vi "ChangePassword-Window.vi"(8 "error in (no error)":errorcluster, 11 "User Info":T1={"UserName"="", "Password"="", "Role"=enum."Admin"}) -> (0 "error out":errorcluster)   [LabVIEW 2017, in "Login-UI.lvlib"]
uses:
  Login-UI.lvlib
  User-Info.ctl
  User-Role.ctl
panel:
  in  "Cancel":bool
  in  "OK":bool
  in  "Password":string="admin" caption="密 码"
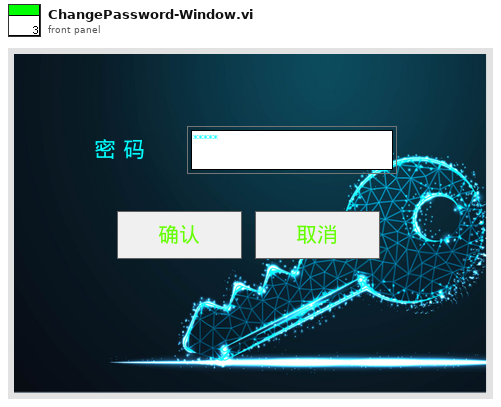
[diagram p1: front panel]
types:
  T1 = typedef "Login-UI.lvlib/User-Info.ctl" = cluster{"UserName":string, "Password":string, "Role":T2}
  T2 = typedef "Login-UI.lvlib/User-Role.ctl" = enum16{"INVALID", "Operator", "Engineer", "Admin"}
  T3 = enum32{"Invalid", "Standard", "Closed", "Hidden", "Minimized", "Maximized"}
  T4 = enum32{"invalid app kind", "Development System", "Run Time System", "Student Edition", "Embedded LabVIEW", "Evaluation", "Custom"}
  T5 = cluster{"Core":cluster{"Current VI Reference":refnum<vi>, "Close Panel on Exit?":bool}, "Your Boolean data":bool, "Your string data":string, "User Info":T1}
  T6 = cluster{"Current VI Reference":refnum<vi>, "Close Panel on Exit?":bool}
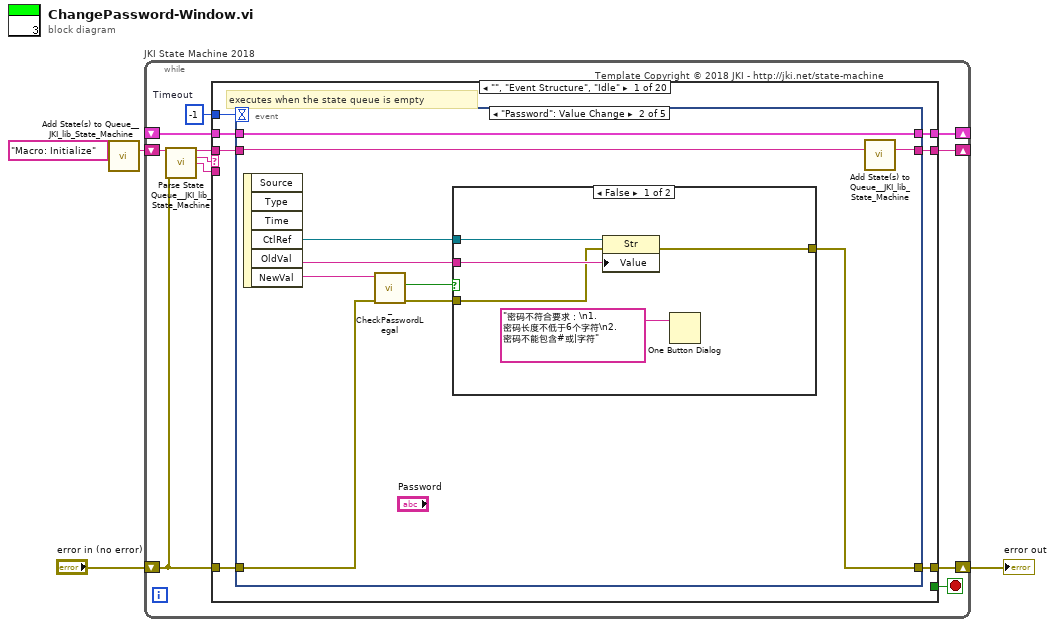
[diagram p0: block diagram]
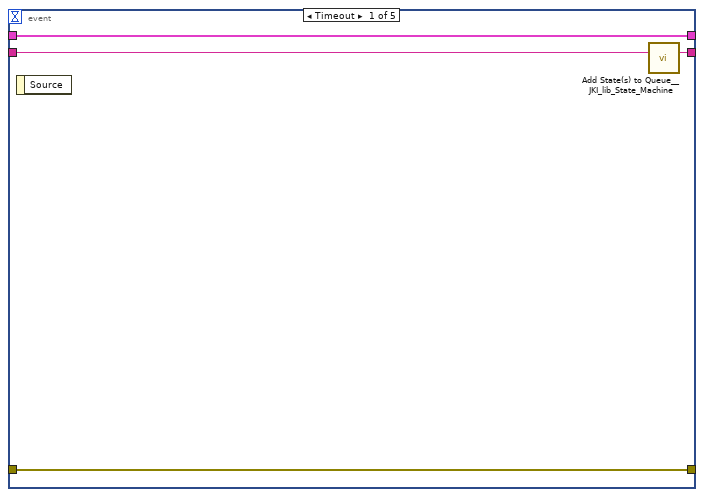
[diagram p2: hidden frame]
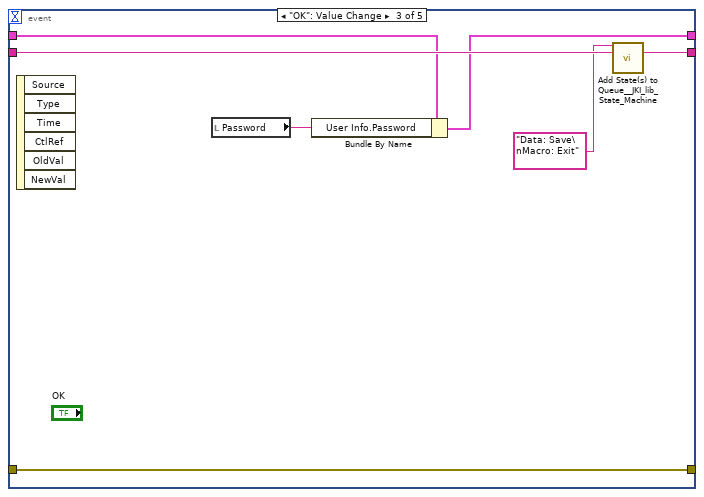
[diagram p4: hidden frame]
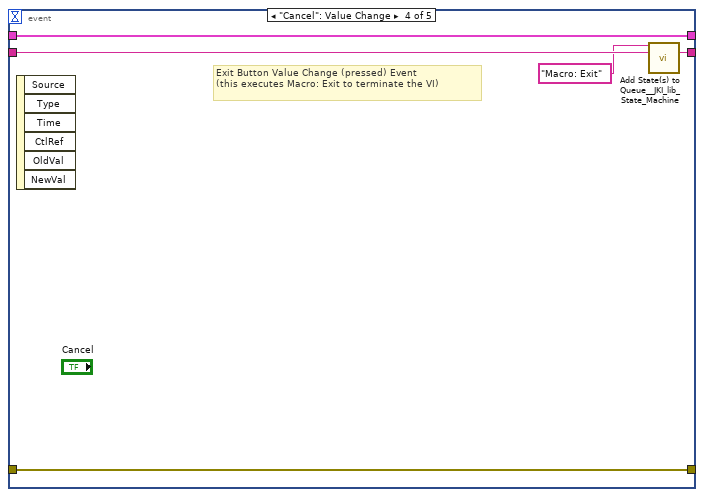
[diagram p5: hidden frame]
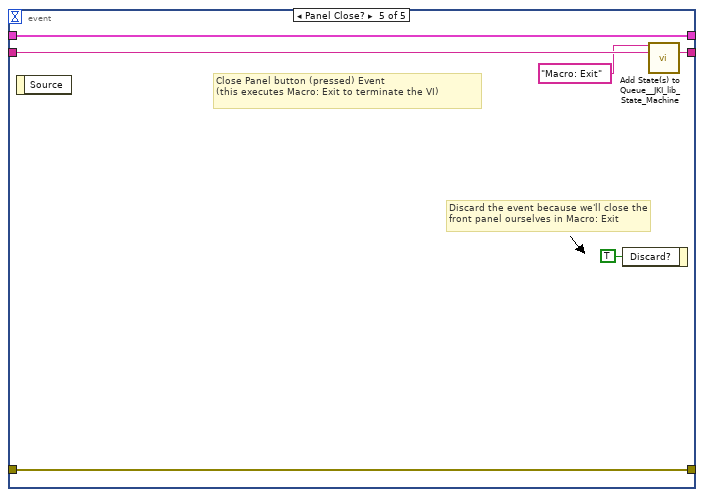
[diagram p6: hidden frame]
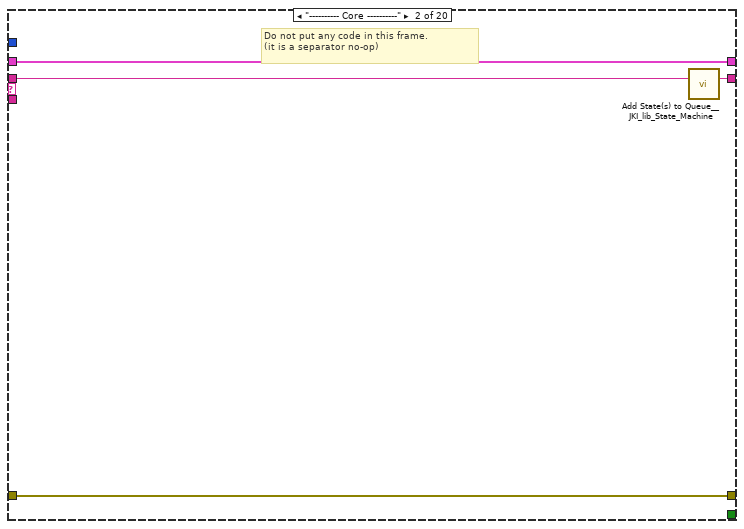
[diagram p7: hidden frame]
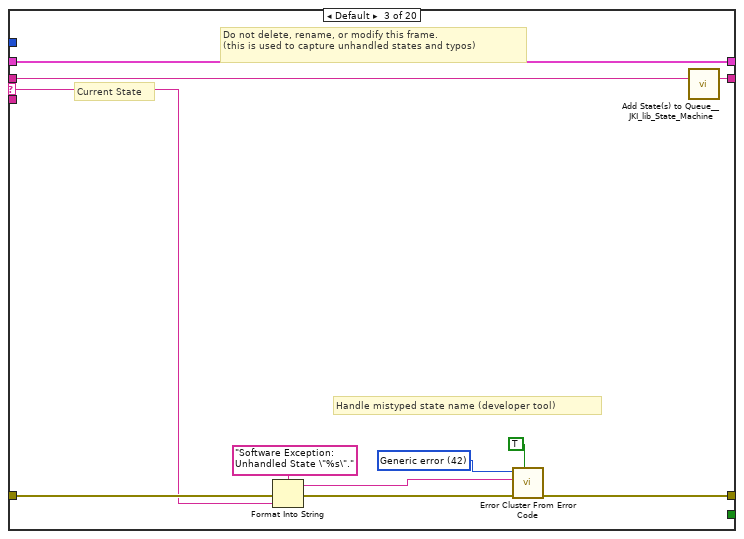
[diagram p8: hidden frame]
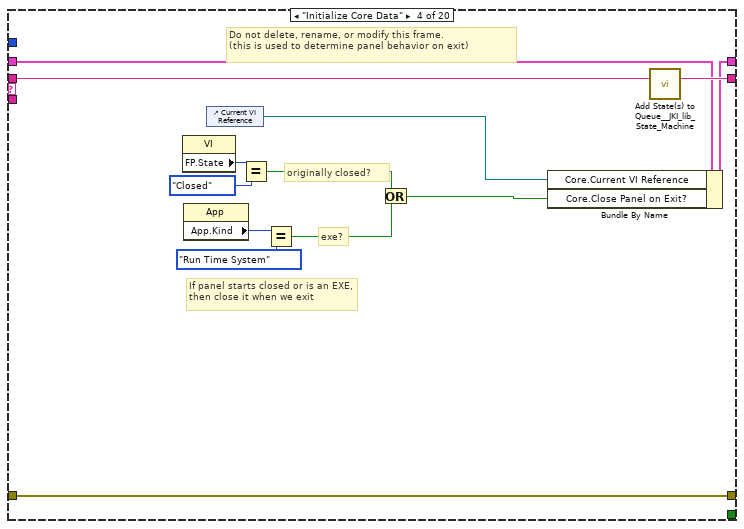
[diagram p9: hidden frame]
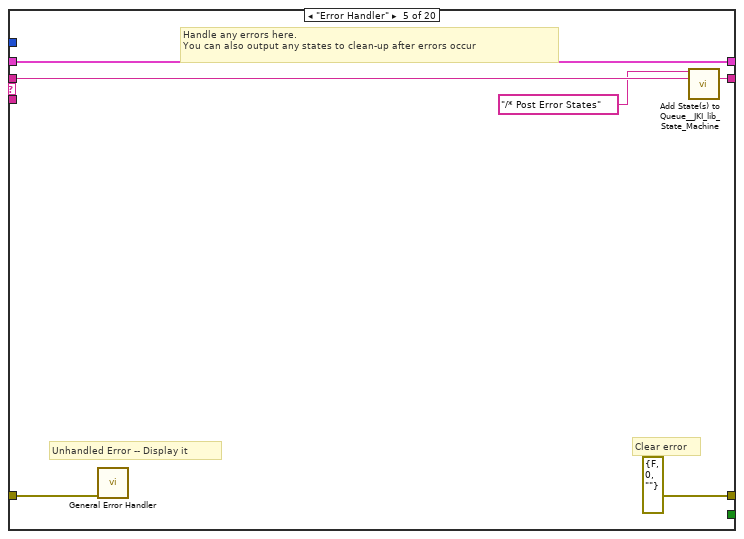
[diagram p10: hidden frame]
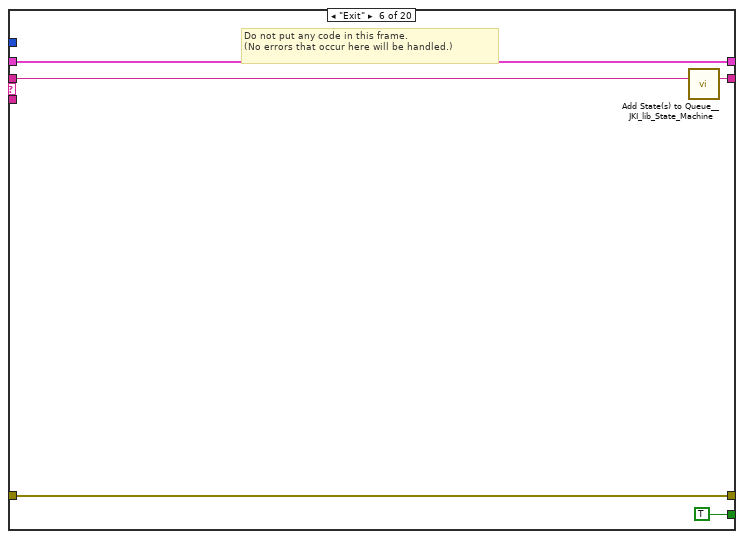
[diagram p11: hidden frame]
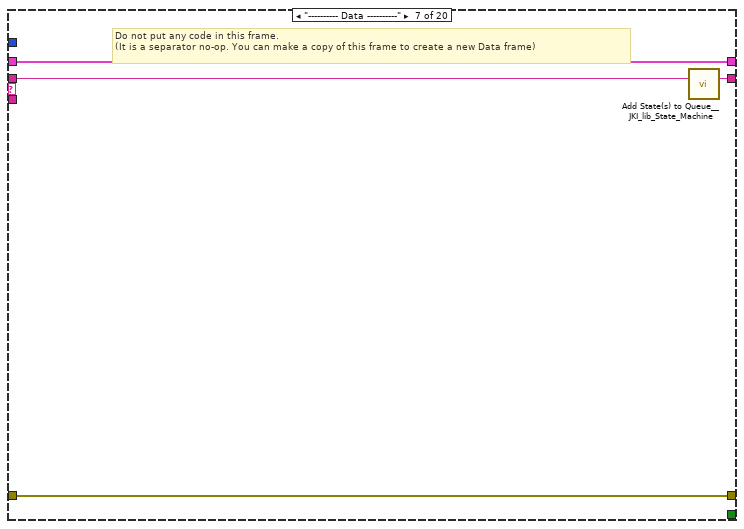
[diagram p12: hidden frame]
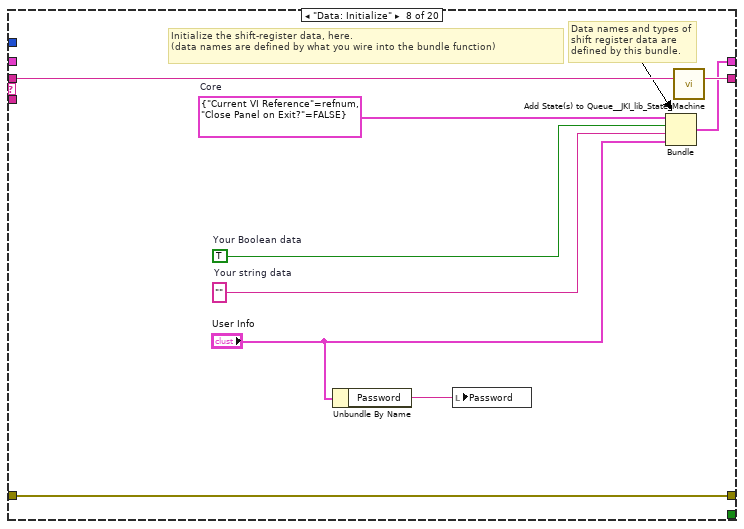
[diagram p13: hidden frame]
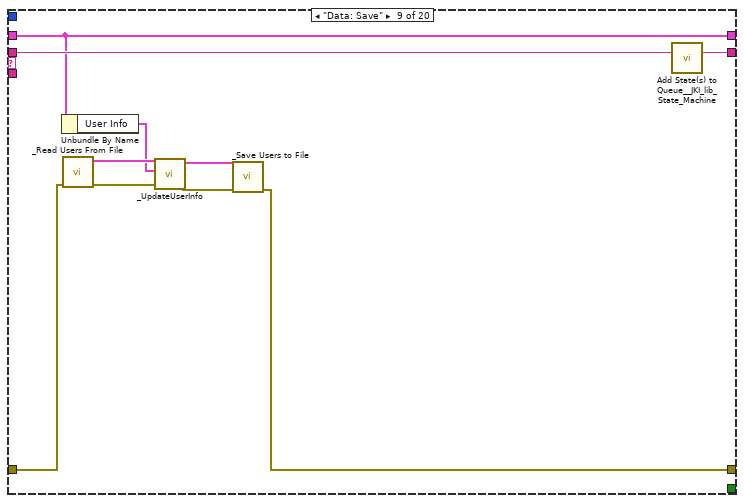
[diagram p14: hidden frame]
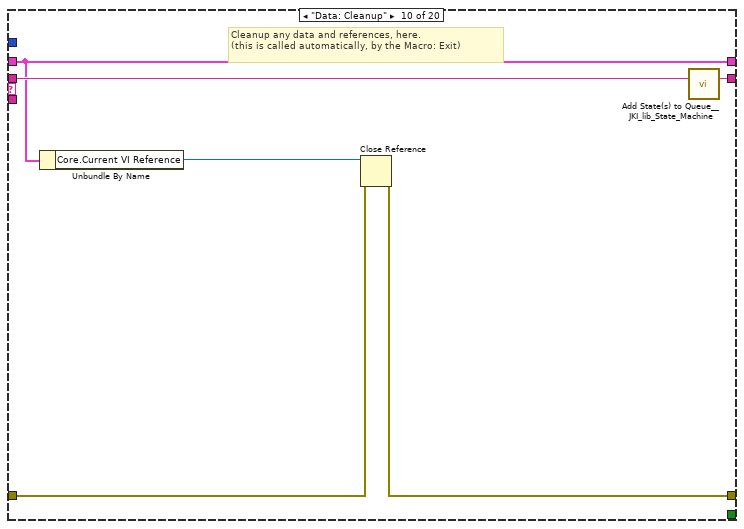
[diagram p15: hidden frame]
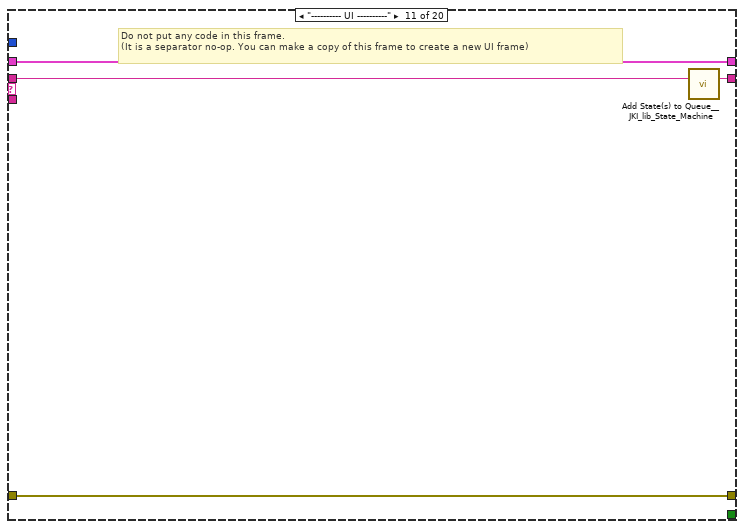
[diagram p16: hidden frame]
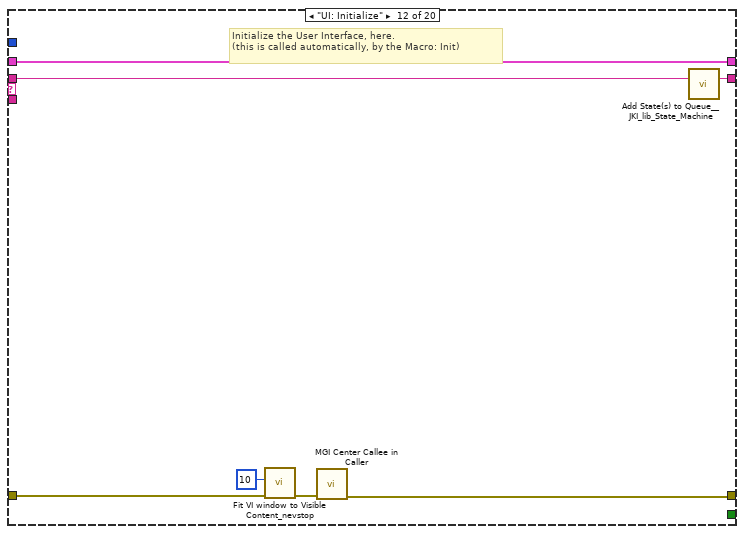
[diagram p17: hidden frame]
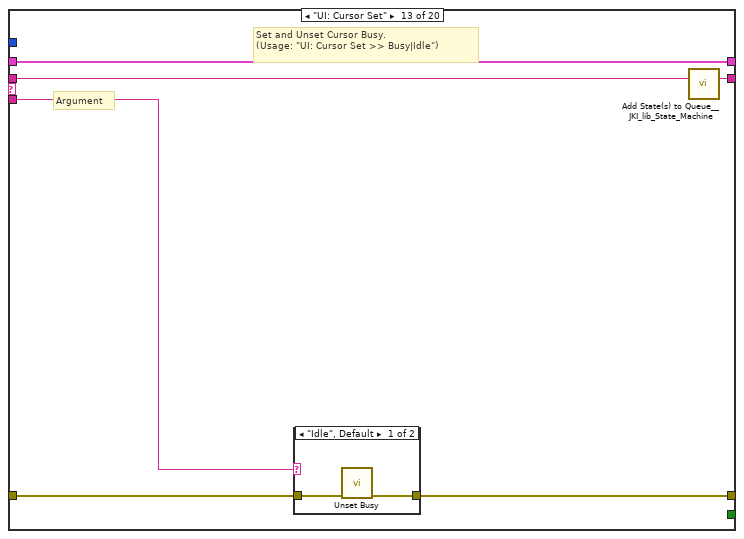
[diagram p18: hidden frame]
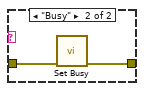
[diagram p19: hidden frame]
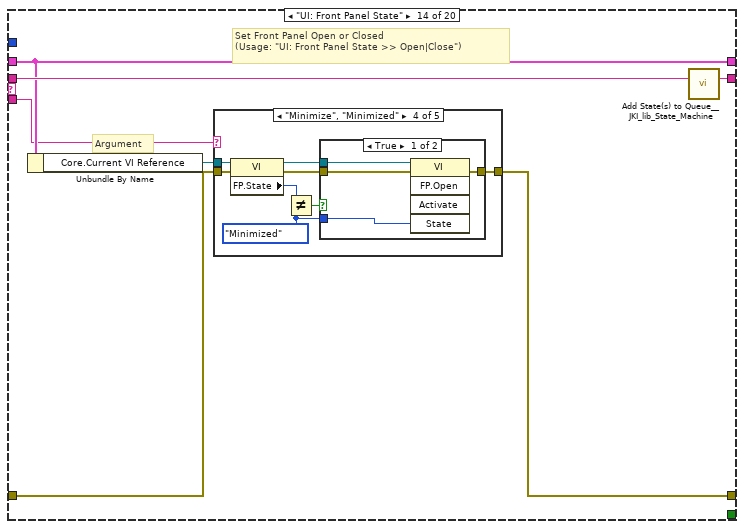
[diagram p20: hidden frame]
diagram:
  n1 = call <vilib>:"Add State(s) to Queue__JKI_lib_State_Machine.vi"("State(s) in (\"\")"="Macro: Initialize") -> ("States Out"=w4:string)  [unwired: 14 in]
  n2 = while "JKI State Machine 2018" {
    shift-right: [w8] -> _
    shift-left: _ -> [w7]
    shift-right: [w11] -> w1
    shift-left: "error in (no error)" -> [w5]
    shift-right: [w10] -> _
    shift-left: w4 -> [w12]
    stop <- w9 stop-if-true
    w6 = -1  # Timeout
    # "Template Copyright © 2018 JKI - http://jki.net/state-machine"
    n3 = call <vilib>:"Parse State Queue__JKI_lib_State_Machine.vi"("State Queue"=w12, "Error In (no error)"=w5) -> ("Remaining States"=w14:string, "Current State"=w15:string, "Arguments"=w13:string)  [unwired: 11 in]
    n4 = case shown="\"\", \"Event Structure\", \"Idle\"" w15 {
      selector: w15 -> [_ _ w65 _ _ _ _ _ _ _ _ _ _ _ _ _ _ _ _ _]
      tunnel: w14 -> [w22 w64 w69 w88 w94 w99 w103 w112 w121 w128 w132 w139 w145 w156 w225 w230 w240 w244 w248 w252]
      tunnel: w13 -> [_ _ _ _ _ _ _ _ _ _ _ _ w140 w150 _ _ _ _ _ _]
      tunnel: w7 -> [w20 w61 w67 w81 w91 w97 w100 _ w113 w123 w129 w137 w143 w152 w222 w227 w237 w241 w245 w249]
      tunnel: [w19 w62 w71 w85 errorcluster {"status"=FALSE, "code"=0, "source"=""} ("error out") w96 w101 w109 w114 w124 w130 w133 w141 w153 w223 w228 w238 w242 w246 w250] -> w11
      tunnel: w5 -> [w18 w62 w70 w85 w90 w96 w101 w109 w115 w125 w130 w134 w142 w154 w223 w228 w238 w242 w246 w250]
      tunnel: [w21 w63 w68 w87 w93 w98 w102 w111 w122 w127 w131 w138 w144 w155 w224 w229 w239 w243 w247 w251] -> w10
      tunnel: [_ _ _ _ _ TRUE _ _ _ _ _ _ _ _ _ _ _ _ _ _] -> w9
      tunnel: [w17 w61 w67 w86 w91 w97 w100 w110 w113 w123 w129 w137 w143 w152 w222 w227 w237 w241 w245 w249] -> w8
      tunnel: w6 -> [w16 _ _ _ _ _ _ _ _ _ _ _ _ _ _ _ _ _ _ _]
      frame "", "Event Structure", "Idle" {
        # "executes when the state queue is empty"
        n5 = event shown="[1] \"Password\": Value Change" {
          selector: _ -> [_ _ _ _ _]
          dyn-events: _ -> [_ _ _ _ _]
          timeout: w16 -> [_ _ _ _ _]
          tunnel: w22 -> [w26 w30 w48 w54 w60]
          tunnel: [w25 w31 w49 w53 w59] -> w21
          tunnel: w20 -> [w23 w32 w46 w51 w57]
          tunnel: [w24 w27 w44 w52 w58] -> w19
          tunnel: w18 -> [w24 w29 w44 w52 w58]
          tunnel: [w23 w32 w45 w51 w57] -> w17
          event Timeout {
            n6 = event-data() -> ()  [unwired: 1 in, 1 out]
            n7 = call <vilib>:"Add State(s) to Queue__JKI_lib_State_Machine.vi"("State(s) in (\"\")"=w26) -> ("States Out"=w25:string)  [unwired: 14 in]
          }
          event "Password": Value Change {
            n8 = event-data() -> ("CtlRef"=w34:refnum<vi>, "OldVal"=w33:string, "NewVal"=w36:string)  [unwired: 1 in, 3 out]
            n9 = call "_CheckPasswordLegal.vi"("error in (no error)"=w29, "Password"=w36) -> ("error out"=w28:errorcluster, "legal?"=w35:bool)  [unwired: 8 in]
            n10 = case shown="False" w35 {
              tunnel: w34 -> [w41 _]
              tunnel: w33 -> [w40 _]
              tunnel: w28 -> [w38 w42]
              tunnel: [w37 w42] -> w27
              frame False {
                n11 = property class="Str"(reference=w41, error in=w38, "Value"=w40) -> (error out=w37:errorcluster)  [unwired: 1 out]
                n12 = One Button Dialog(message="密码不符合要求：\n1.密码长度不低于6个字符\n2. 密码不能包含#或|字符") -> ()  [unwired: 1 in, 1 out]
              }
              frame True {
              }
            }
            n13 = call <vilib>:"Add State(s) to Queue__JKI_lib_State_Machine.vi"("State(s) in (\"\")"=w30) -> ("States Out"=w31:string)  [unwired: 14 in]
          }
          event "OK": Value Change {
            n14 = event-data() -> ()  [unwired: 1 in, 6 out]
            n15 = local read "Password"() -> (w43:string)
            n16 = Bundle By Name(cluster=w46, "User Info.Password"=w43) -> (w45:T5)
            n17 = call <vilib>:"Add State(s) to Queue__JKI_lib_State_Machine.vi"("State(s) in Front (\"\")"="Data: Save\nMacro: Exit", "State(s) in (\"\")"=w48) -> ("States Out"=w49:string)  [unwired: 13 in]
          }
          event "Cancel": Value Change {
            # "Exit Button Value Change (pressed) Event\n(this executes Macro: Exit to terminate the VI)"
            n18 = event-data() -> ()  [unwired: 1 in, 6 out]
            n19 = call <vilib>:"Add State(s) to Queue__JKI_lib_State_Machine.vi"("State(s) in Front (\"\")"="Macro: Exit", "State(s) in (\"\")"=w54) -> ("States Out"=w53:string)  [unwired: 13 in]
          }
          event Panel Close? {
            # "Discard the event because we'll close the front panel ourselves in Macro: Exit"
            # "Close Panel button (pressed) Event\n(this executes Macro: Exit to terminate the VI)"
            n20 = event-data() -> ()  [unwired: 1 in, 1 out]
            n21 = event-data("Discard?"=TRUE) -> ()  [unwired: 1 in, 1 out]
            n22 = call <vilib>:"Add State(s) to Queue__JKI_lib_State_Machine.vi"("State(s) in Front (\"\")"="Macro: Exit", "State(s) in (\"\")"=w60) -> ("States Out"=w59:string)  [unwired: 13 in]
          }
        }
      }
      frame "---------- Core ----------" {
        # "Do not put any code in this frame.\n(it is a separator no-op)"
        n23 = call <vilib>:"Add State(s) to Queue__JKI_lib_State_Machine.vi"("State(s) in (\"\")"=w64) -> ("States Out"=w63:string)  [unwired: 14 in]
      }
      frame Default {
        w74 = 42 items=["No error", "Argument error", "Memory is full", "Out of zone", "End of file", "File already open", "Generic file I/O error", "File not found", "File permission error", "Disk is full", "Duplicate path", "Too many files open", "System feature not enabled", "Resource file not found", "Cannot add resource", "Resource not found", "Image not found", "Image memory error", "Pen does not exist", "Config type invalid", "Config token not found", "Config parse error", "Config memory error", "Bad external code format", "Bad external code offset", "External code not present", "Null window", "Destroy window error", "Null menu", "Print aborted", "Bad print record", "Print driver error", "Windows error during printing", "Memory error during printing", "Print dialog error", "Generic print error", "Invalid device refnum", "Device not found", "Device parameter error", "Device unit error", "Cannot open device", "Device call aborted", "Generic error", "Cancelled by user", "Object ID too low", "Object ID too high", "Object not in heap", "Unknown heap", "Unknown object (invalid DefProc)", "Unknown object (DefProc not in table)", "Message out of range", "Invalid (null) method", "Unknown message", "Manager call not supported", "Bad address", "Network operation in progress", "Network operation timed out", "Connection is busy", "Network attribute not supported", "Network error", "Address in use", "System out of memory", "Connection aborted", "Connection refused", "Not connected", "Already connected", "Connection closed", "Initialization error (interapplication manager)", "Bad occurrence", "Wait on unbound occurrence handler", "Occurrence queue overflow", "Datalog type conflict", "Unused", "Unrecognized type (interapplication manager)", "Memory corrupt", "Failed to make temporary DLL", "Old CIN version", "Drag socket not found", "Failed to load drop-object", "Failed to register OLE object", "Failed to release OLE object", "Format specifier type mismatch", "Unknown format specifier", "Too few format specifiers", "Too many format specifiers", "Scan failed", "Newer CIN version", "Error converting to variant", "Runtime menu error", "Password tampered", "Variant attribute not found", "Incompatible variant data type", "Event data is not available", "Event Store is not present", "Occurrence is not found", "Event Queue is not created", "Event info is not available", "Refnum passed is NULL", "Error retrieving Class GUID", "Error retrieving CoClass GUID", "Error retrieving TypeLib GUID.", "Bad built application magic bytes.", "Specific driver is different from the specific driver associated with the Logical Name.", "There is no session opened to the class driver.", "Max Error", "MAX - Error with config objects", "MAX - Error loading configuration", "MAX - Group not supported"]
        # "Current State"
        # "Do not delete, rename, or modify this frame.\n(this is used to capture unhandled states and typos)"
        # "Handle mistyped state name (developer tool)"
        n24 = Format Into String(format string="Software Exception: Unhandled State \"%s\"." ("message"), error in=w70, w65) -> (resulting string=w73:string, error out=w72:errorcluster)  [unwired: 1 in]
        n25 = call <vilib>:"Error Cluster From Error Code.vi"("show call chain? (False)"=TRUE, "error in (no error)"=w72, "error message (\"\")"=w73, "error code (0)"=w74) -> ("error out"=w71:errorcluster)  [unwired: 5 in]
        n26 = call <vilib>:"Add State(s) to Queue__JKI_lib_State_Machine.vi"("State(s) in (\"\")"=w69) -> ("States Out"=w68:string)  [unwired: 14 in]
      }
      frame "Initialize Core Data" {
        # "Do not delete, rename, or modify this frame.\n(this is used to determine panel behavior on exit)"
        # "originally closed?"
        # "exe?"
        # "If panel starts closed or is an EXE, then close it when we exit"
        n27 = property class="VI"() -> ("FP.State"=w78:T3)  [unwired: 2 in, 2 out]
        n28 = property class="App"() -> ("App.Kind"=w84:T4)  [unwired: 2 in, 2 out]
        n29 = control-ref of="Current VI Reference"() -> (w79:refnum<vi>)
        n30 = Equal?(x=w78, y=T3."Closed" ("Front Panel Window:State")) -> (x = y?=w76:bool)
        n31 = Equal?(x=w84, y=T4."Run Time System" ("Application:Kind")) -> (x = y?=w82:bool)
        n32 = Or(x=w76, y=w82) -> (x .or. y?=w80:bool)
        n33 = Bundle By Name(cluster=w81, "Core.Current VI Reference"=w79, "Core.Close Panel on Exit?"=w80) -> (w86:T5)
        n34 = call <vilib>:"Add State(s) to Queue__JKI_lib_State_Machine.vi"("State(s) in (\"\")"=w88) -> ("States Out"=w87:string)  [unwired: 14 in]
      }
      frame "Error Handler" {
        # "Unhandled Error -- Display it"
        # "Handle any errors here.\nYou can also output any states to clean-up after errors occur"
        # "Clear error"
        n35 = call <vilib>:"General Error Handler.vi"("error in (no error)"=w90) -> ()  [unwired: 10 in, 5 out]
        n36 = call <vilib>:"Add State(s) to Queue__JKI_lib_State_Machine.vi"("State(s) in Front (\"\")"="/* Post Error States", "State(s) in (\"\")"=w94) -> ("States Out"=w93:string)  [unwired: 13 in]
      }
      frame "Exit" {
        # "Do not put any code in this frame.\n(No errors that occur here will be handled.)"
        n37 = call <vilib>:"Add State(s) to Queue__JKI_lib_State_Machine.vi"("State(s) in (\"\")"=w99) -> ("States Out"=w98:string)  [unwired: 14 in]
      }
      frame "---------- Data ----------" {
        # "Do not put any code in this frame.\n(It is a separator no-op. You can make a copy of this frame to create a new Data frame)"
        n38 = call <vilib>:"Add State(s) to Queue__JKI_lib_State_Machine.vi"("State(s) in (\"\")"=w103) -> ("States Out"=w102:string)  [unwired: 14 in]
      }
      frame "Data: Initialize" {
        w106 = T6 {"Current VI Reference"=refnum, "Close Panel on Exit?"=FALSE}  # Core
        w108 = TRUE  # Your Boolean data
        w107 = ""  # Your string data
        # "Data names and types of shift register data are defined by this bundle."
        # "Initialize the shift-register data, here.\n(data names are defined by what you wire into the bundle function)"
        n39 = Unbundle By Name("User Info") -> ("Password"=w104:string)
        n40 = local write "Password"(w104) -> ()
        n41 = Bundle("Core"=w106, "Your Boolean data"=w108, "Your string data"=w107, "User Info"="User Info") -> (w110:T5)  [unwired: 1 in]
        n42 = call <vilib>:"Add State(s) to Queue__JKI_lib_State_Machine.vi"("State(s) in (\"\")"=w112) -> ("States Out"=w111:string)  [unwired: 14 in]
      }
      frame "Data: Save" {
        n43 = Unbundle By Name(w113) -> ("User Info"=w119:T1)
        n44 = call "_Read Users From File.vi"("Error in"=w115) -> ("Error out"=w118:errorcluster, "Array"=w120:T1[])  [unwired: 9 in]
        n45 = call "_UpdateUserInfo.vi"("error in"=w118, "User"=w119, "User List"=w120) -> ("error out"=w116:errorcluster, "User List"=w117:T1[])  [unwired: 7 in]
        n46 = call "_Save Users to File.vi"("Error in"=w116, "Array"=w117) -> ("Error out"=w114:errorcluster)  [unwired: 9 in]
        n47 = call <vilib>:"Add State(s) to Queue__JKI_lib_State_Machine.vi"("State(s) in (\"\")"=w121) -> ("States Out"=w122:string)  [unwired: 14 in]
      }
      frame "Data: Cleanup" {
        # "Cleanup any data and references, here.\n(this is called automatically, by the Macro: Exit)"
        n48 = Unbundle By Name(w123) -> ("Core.Current VI Reference"=w126:refnum<vi>)
        n49 = Close Reference(reference=w126, error in (no error)=w125) -> (error out=w124:errorcluster)
        n50 = call <vilib>:"Add State(s) to Queue__JKI_lib_State_Machine.vi"("State(s) in (\"\")"=w128) -> ("States Out"=w127:string)  [unwired: 14 in]
      }
      frame "---------- UI ----------" {
        # "Do not put any code in this frame.\n(It is a separator no-op. You can make a copy of this frame to create a new UI frame)"
        n51 = call <vilib>:"Add State(s) to Queue__JKI_lib_State_Machine.vi"("State(s) in (\"\")"=w132) -> ("States Out"=w131:string)  [unwired: 14 in]
      }
      frame "UI: Initialize" {
        # "Initialize the User Interface, here.\n(this is called automatically, by the Macro: Init)"
        n52 = call <userlib>:"Fit VI window to Visible Content_nevstop.vi"("error in (no error)"=w134, "border spacing (2 px)"=10) -> ("error out"=w136:errorcluster)  [unwired: 4 in, 1 out]
        n53 = call <userlib>:"MGI Center Callee in Caller.vi"("Error In"=w136) -> ("Error Out"=w133:errorcluster)  [unwired: 10 in]
        n54 = call <vilib>:"Add State(s) to Queue__JKI_lib_State_Machine.vi"("State(s) in (\"\")"=w139) -> ("States Out"=w138:string)  [unwired: 14 in]
      }
      frame "UI: Cursor Set" {
        # "Argument"
        # "Set and Unset Cursor Busy.\n(Usage: \"UI: Cursor Set >> Busy|Idle\")"
        n55 = case shown="\"Idle\", Default" w140 {
          tunnel: w142 -> [w147 w149]
          tunnel: [w146 w148] -> w141
          frame "Idle", Default {
            n56 = call <vilib>:"Unset Busy.vi"("error in (no error)"=w147) -> ("error out"=w146:errorcluster)  [unwired: 10 in]
          }
          frame "Busy" {
            n57 = call <vilib>:"Set Busy.vi"("error in (no error)"=w149) -> ("error out"=w148:errorcluster)  [unwired: 9 in, 1 out]
          }
        }
        n58 = call <vilib>:"Add State(s) to Queue__JKI_lib_State_Machine.vi"("State(s) in (\"\")"=w145) -> ("States Out"=w144:string)  [unwired: 14 in]
      }
      frame "UI: Front Panel State" {
        # "Argument"
        # "Set Front Panel Open or Closed\n(Usage: \"UI: Front Panel State >> Open|Close\")"
        n59 = Unbundle By Name(w152) -> ("Core.Current VI Reference"=w151:refnum<vi>)
        n60 = case shown="\"Minimize\", \"Minimized\"" w150 {
          tunnel: w154 -> [w162 w177 w188 w201 w214]
          tunnel: [w164 w178 w190 w203 w216] -> w153
          tunnel: w151 -> [w163 w175 w189 w202 w215]
          frame "Open", "Standard", Default {
            w157 = T3."Standard" ("State")
            n61 = property class="VI"(reference=w163, error in=w162) -> (reference out=w160:refnum<vi>, error out=w161:errorcluster, "FP.State"=w159:T3)
            n62 = Not Equal?(x=w159, y=w157) -> (x != y?=w158:bool)
            n63 = case shown="True" w158 {
              tunnel: [w168 w170] -> w164
              tunnel: w161 -> [w167 w170]
              tunnel: w160 -> [w166 _]
              tunnel: w157 -> [w165 _]
              frame True {
                n64 = invoke class="VI" method="FP.Open"(reference=w166, error in=w167, "Activate"=TRUE, "State"=w165) -> (error out=w168:errorcluster)  [unwired: 1 in, 4 out]
              }
              frame False {
              }
            }
          }
          frame "Close", "Closed" {
            n65 = property class="VI"(reference=w175, error in=w177) -> (reference out=w174:refnum<vi>, error out=w176:errorcluster, "FP.State"=w172:T3)
            n66 = Not Equal?(x=w172, y=T3."Closed" ("Front Panel Window:State")) -> (x != y?=w171:bool)
            n67 = case shown="True" w171 {
              tunnel: [w179 w182] -> w178
              tunnel: w176 -> [w179 w181]
              tunnel: w174 -> [_ w180]
              frame False {
              }
              frame True {
                n68 = invoke class="VI" method="FP.Close"(reference=w180, error in=w181) -> (error out=w182:errorcluster)  [unwired: 1 in, 2 out]
              }
            }
          }
          frame "Hidden", "Hide" {
            w183 = T3."Hidden" ("State")
            n69 = property class="VI"(reference=w189, error in=w188) -> (reference out=w186:refnum<vi>, error out=w187:errorcluster, "FP.State"=w185:T3)
            n70 = Not Equal?(x=w185, y=w183) -> (x != y?=w184:bool)
            n71 = case shown="True" w184 {
              tunnel: [w194 w195] -> w190
              tunnel: w187 -> [w193 w195]
              tunnel: w186 -> [w192 _]
              tunnel: w183 -> [w191 _]
              frame True {
                n72 = invoke class="VI" method="FP.Open"(reference=w192, error in=w193, "State"=w191) -> (error out=w194:errorcluster)  [unwired: 2 in, 4 out]
              }
              frame False {
              }
            }
          }
          frame "Minimize", "Minimized" {
            w196 = T3."Minimized" ("State")
            n73 = property class="VI"(reference=w202, error in=w201) -> (reference out=w199:refnum<vi>, error out=w200:errorcluster, "FP.State"=w198:T3)
            n74 = Not Equal?(x=w198, y=w196) -> (x != y?=w197:bool)
            n75 = case shown="True" w197 {
              tunnel: [w207 w208] -> w203
              tunnel: w200 -> [w206 w208]
              tunnel: w199 -> [w205 _]
              tunnel: w196 -> [w204 _]
              frame True {
                n76 = invoke class="VI" method="FP.Open"(reference=w205, error in=w206, "State"=w204) -> (error out=w207:errorcluster)  [unwired: 2 in, 4 out]
              }
              frame False {
              }
            }
          }
          frame "Maximize", "Maximized" {
            w209 = T3."Maximized" ("State")
            n77 = property class="VI"(reference=w215, error in=w214) -> (reference out=w212:refnum<vi>, error out=w213:errorcluster, "FP.State"=w211:T3)
            n78 = Not Equal?(x=w211, y=w209) -> (x != y?=w210:bool)
            n79 = case shown="True" w210 {
              tunnel: [w220 w221] -> w216
              tunnel: w213 -> [w219 w221]
              tunnel: w212 -> [w218 _]
              tunnel: w209 -> [w217 _]
              frame True {
                n80 = invoke class="VI" method="FP.Open"(reference=w218, error in=w219, "State"=w217) -> (error out=w220:errorcluster)  [unwired: 2 in, 4 out]
              }
              frame False {
              }
            }
          }
        }
        n81 = call <vilib>:"Add State(s) to Queue__JKI_lib_State_Machine.vi"("State(s) in (\"\")"=w156) -> ("States Out"=w155:string)  [unwired: 14 in]
      }
      frame "---------- Macro ----------" {
        # "Do not put any code in this frame.\n(It is a separator no-op. You can make a copy of this frame to create a new Macro frame)"
        n82 = call <vilib>:"Add State(s) to Queue__JKI_lib_State_Machine.vi"("State(s) in (\"\")"=w225) -> ("States Out"=w224:string)  [unwired: 14 in]
      }
      frame "Macro: Initialize" {
        w226 = "Data: Initialize\nInitialize Core Data\nUI: Initialize\nUI: Front Panel State >> Open"  # Data: Initialize Initialize Core Data UI: Initialize UI: Front Panel State >> Open
        # "Initialization Macro\n(This is called once, when the VI starts)"
        n83 = call <vilib>:"Add State(s) to Queue__JKI_lib_State_Machine.vi"("State(s) in Front (\"\")"=w226, "State(s) in (\"\")"=w230) -> ("States Out"=w229:string)  [unwired: 13 in]
      }
      frame "Macro: Exit" {
        # "Exit Macro\n(This is called once, when the VI exits)"
        n84 = Unbundle By Name(w237) -> ("Core.Close Panel on Exit?"=w236:bool)
        n85 = Select(t="UI: Front Panel State >> Close", s=w236, f="") -> (s? t:f=w233:string)
        n86 = call <vilib>:"Add State(s) to Queue__JKI_lib_State_Machine.vi"("State(s) in (\"\")"=w233, "State(s) at Back (\"\")"="Data: Cleanup\nExit") -> ("States Out"=w231:string)  [unwired: 13 in]
        n87 = call <vilib>:"Add State(s) to Queue__JKI_lib_State_Machine.vi"("State(s) in Front (\"\")"=w231, "State(s) in (\"\")"=w240) -> ("States Out"=w239:string)  [unwired: 13 in]
      }
      frame "---------- New Category ----------" {
        # "Template Separator\n(You can make a copy of, or modify, this frame)"
        n88 = call <vilib>:"Add State(s) to Queue__JKI_lib_State_Machine.vi"("State(s) in (\"\")"=w244) -> ("States Out"=w243:string)  [unwired: 14 in]
      }
      frame "New Category: 1" {
        # "Your code here.\n(You can make a copy of, or modify, this frame)"
        n89 = call <vilib>:"Add State(s) to Queue__JKI_lib_State_Machine.vi"("State(s) in (\"\")"=w248) -> ("States Out"=w247:string)  [unwired: 14 in]
      }
      frame "New Category: 2" {
        # "Your code here.\n(You can make a copy of, or modify, this frame)"
        n90 = call <vilib>:"Add State(s) to Queue__JKI_lib_State_Machine.vi"("State(s) in (\"\")"=w252) -> ("States Out"=w251:string)  [unwired: 14 in]
      }
    }
  }
  "error out" <- w1
